vi "QT_FGCleanUp.vi"(5 "error in (no error)":errorcluster, 8 "Private":T1) -> (19 "error out":errorcluster)   [LabVIEW 2024]
doc: "CleanUp any open Grabbing sessions, use with caution!\nInformation are only displayed in the debug window, set 'Private>Reserved1' to 4 to see what is going on.\n© Ch. Salzmann, 1994-2004"
uses:
  <userlib>/ImageProcessing/QTLIB_2595_LV86/QT_Selector.ctl
  <userlib>/ImageProcessing/QTLIB_2595_LV86/QT_Private.ctl
panel:
  # "CleanUp any open Grabbing sessions, use with caution!\nInformation are only displayed in the debug window, \n                    set 'Private>reserved 1' to 4 to see what is going on.\n© Ch. Salzmann, 1994-2005"
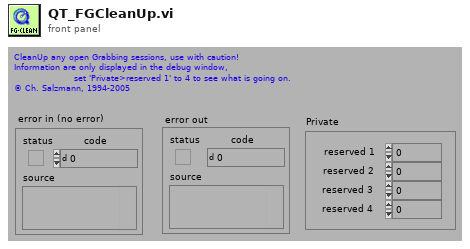
[diagram p1: front panel]
types:
  T1 = typedef "QT_Private.ctl" = cluster{"reserved 1":i32, "reserved 2":i32, "reserved 3":i32, "reserved 4":i32}
  T2 = typedef "QT_Selector.ctl" = enum32{"do nothing", "Get all Sources", "Get Source info", "Open Image", "Save Image to File", "Effect", "Close", "SG Grab", "Compress in Memory", "Decompress to Memory", "New Movie", "Open Movie", "Add Frame", "Get Frame", "Close Movie", "Get QT & CIN info", "SG init", "SG Close", "Open sound file", "Close sound file", "Read sound data", "Write sound data", "Import sound", "Export sound", "Add sound to movie", "Get sound from movie", "reserved", "reserved 1", "reserved 2"}
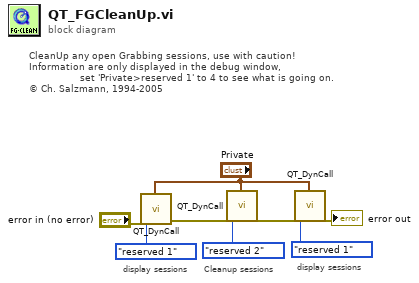
[diagram p0: block diagram]
diagram:
  # "display sessions"
  # "display sessions"
  # "Cleanup sessions"
  # "CleanUp any open Grabbing sessions, use with caution!\nInformation are only displayed in the debug window, \n                 set 'Private>reserved 1' to 4 to see what is going on.\n© Ch. Salzmann, 1994-2005"
  n1 = call <userlib>:"QT_DynCall.vi"("error in (no error)"="error in (no error)", "Selector"=QT_Selector."reserved 1", "Private"="Private") -> ("error out"=w4:errorcluster)  [unwired: 9 in, 15 out]
  n2 = call <userlib>:"QT_DynCall.vi"("error in (no error)"=w4, "Selector"=QT_Selector."reserved 2", "Private"="Private") -> ("error out"=w7:errorcluster)  [unwired: 9 in, 15 out]
  n3 = call <userlib>:"QT_DynCall.vi"("error in (no error)"=w7, "Selector"=QT_Selector."reserved 1", "Private"="Private") -> ("error out"=→"error out":errorcluster)  [unwired: 9 in, 15 out]
